vi "ml.vi"() -> ()   [LabVIEW 2014]
uses:
  ml64i4.dll
panel:
  out "Argument":string="LabVIEW"
  out "Cursor":i32
  in  "Console":string
  in  "Link":enum16{"Kernel", "Install"}(ring)=enum."Install"
  in  "ON":bool
  in  "Quit":bool
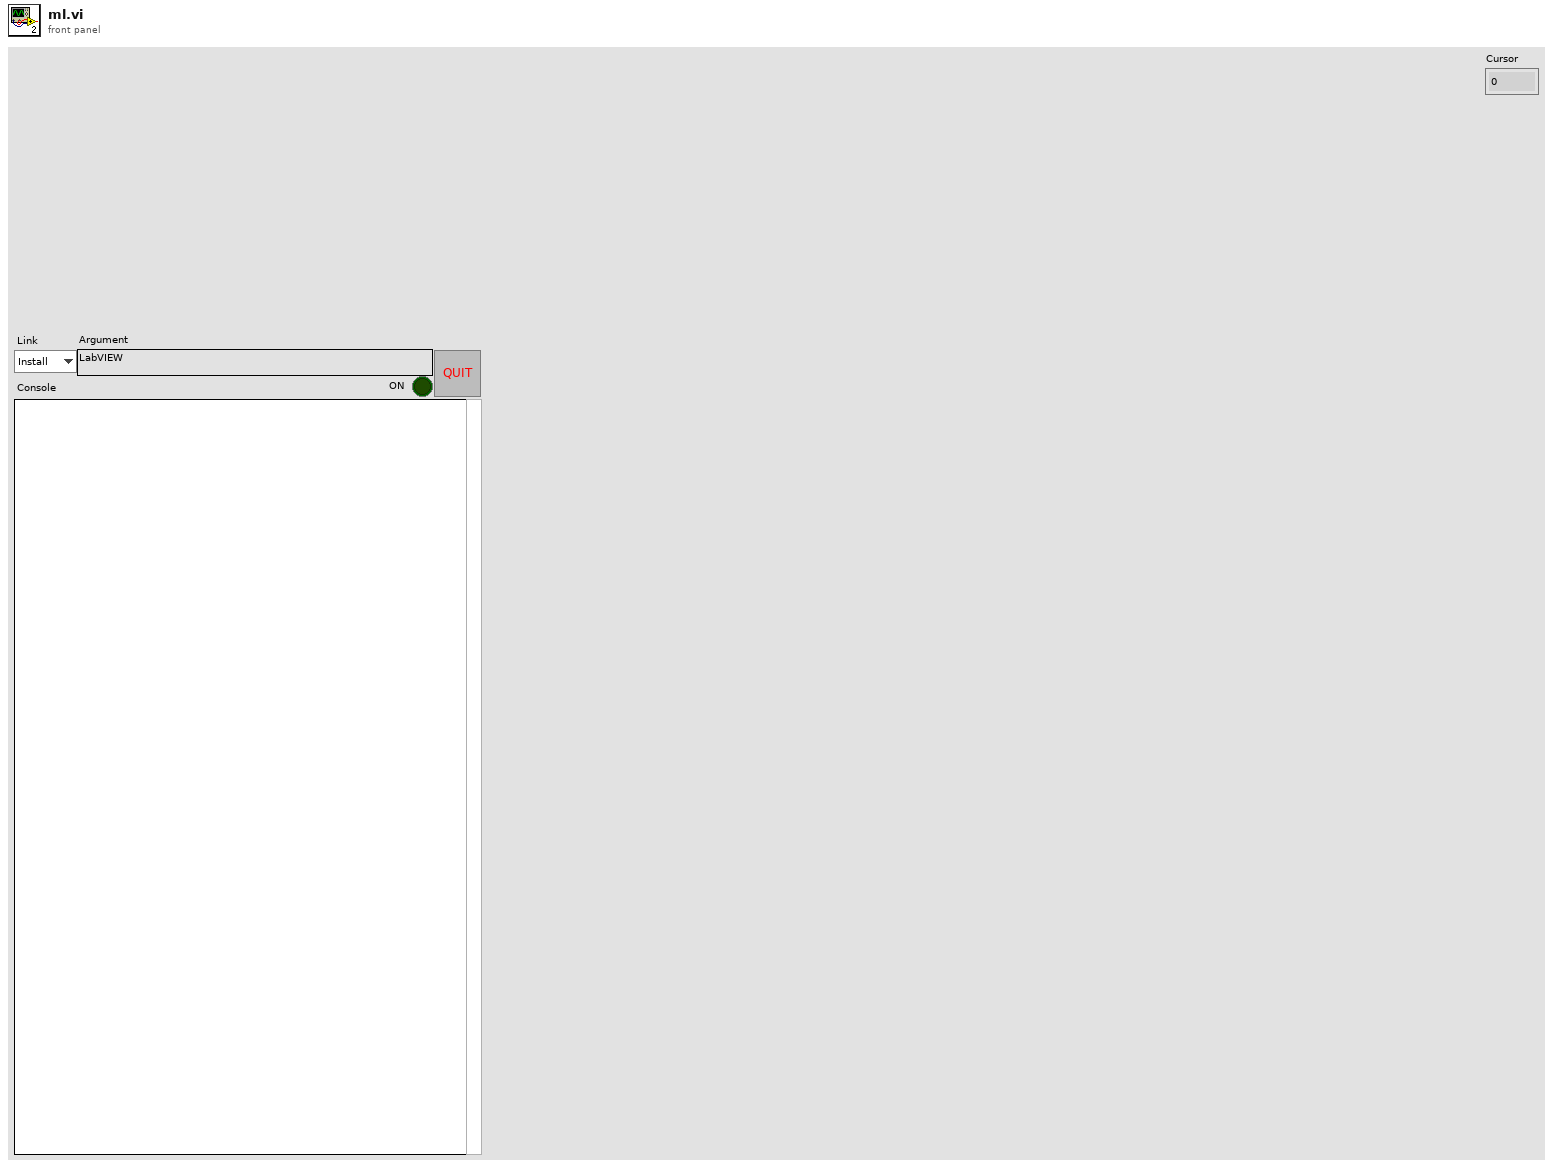
[diagram p1: front panel]
types:
  T1 = typedef "eventvkey.ctl" = enum16{"ASCII", "Enter", "Return", "Shift", "Ctrl", "Alt", "Cmd", "Opt", "Caps", "NumLock", "Clear", "Break", "Up", "Down", "Left", "Right", "Insert", "Delete", "Home", "End", "PageUp", "PageDown", "Escape", "Help", "Pause", "ScrollLock", "F1", "F2", "F3", "F4", "F5", "F6", "F7", "F8", "F9", "F10", "F11", "F12", "F13", "F14", "F15", "F16", "F17", "F18", "F19", "F20", "F21", "F22", "F23", "F24", "Play", "VolumeUp", "VolumeDown", "Mute", "Two Byte Char"}
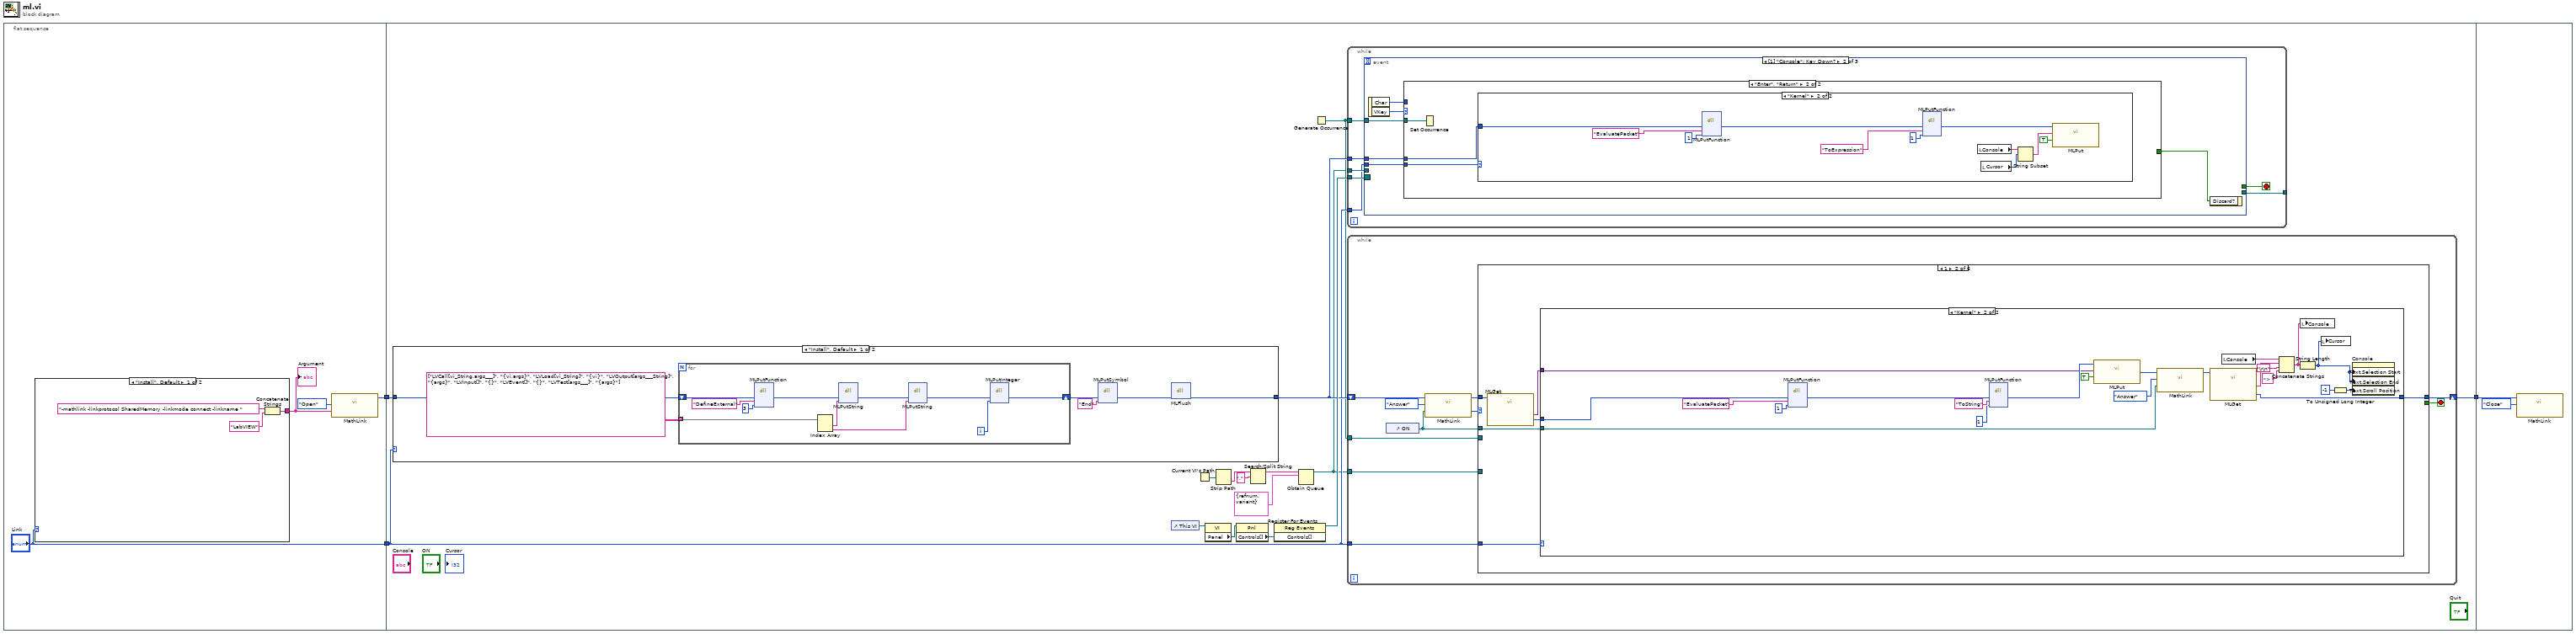
[diagram p0: block diagram]
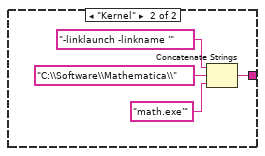
[diagram p2: hidden frame]
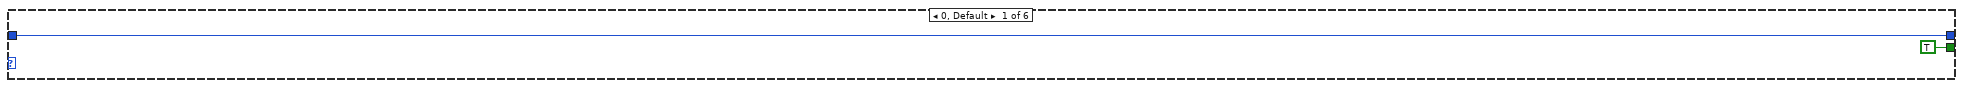
[diagram p3: hidden frame]
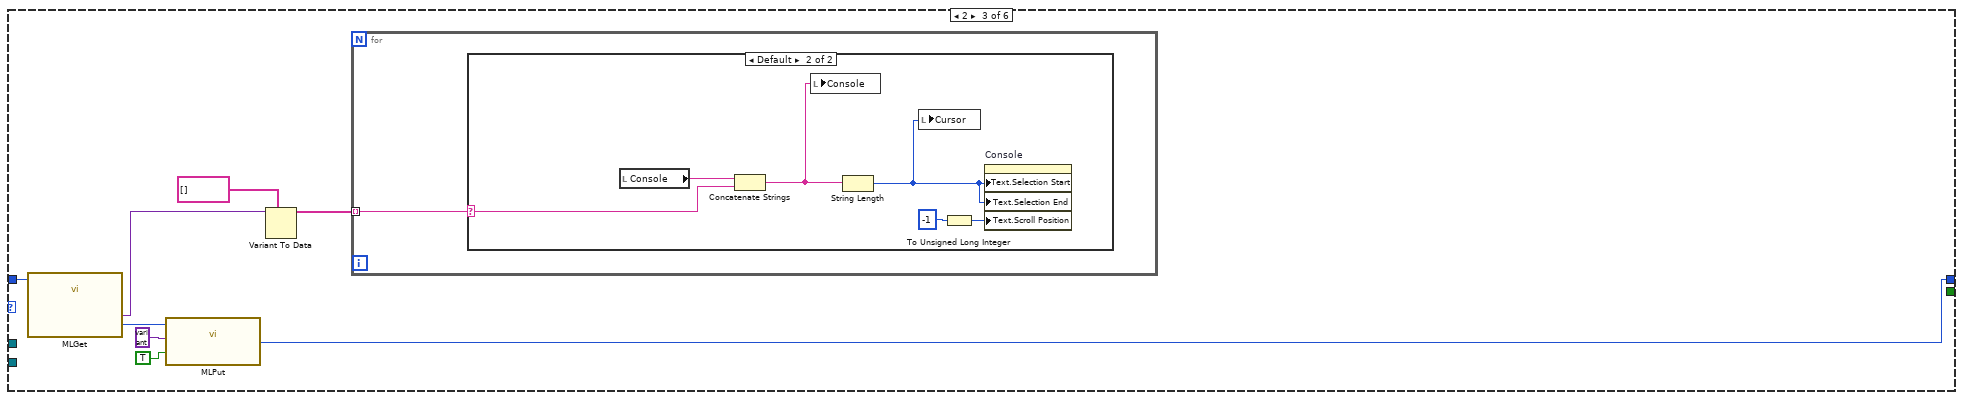
[diagram p5: hidden frame]
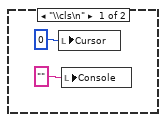
[diagram p6: hidden frame]
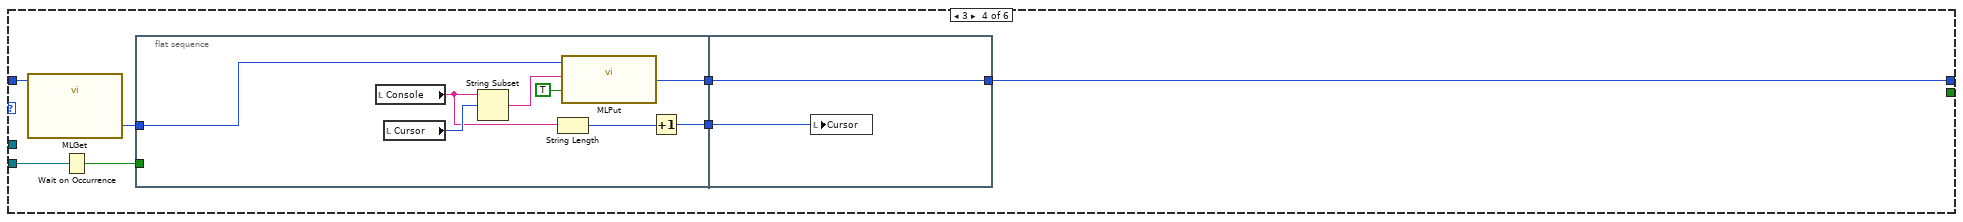
[diagram p7: hidden frame]
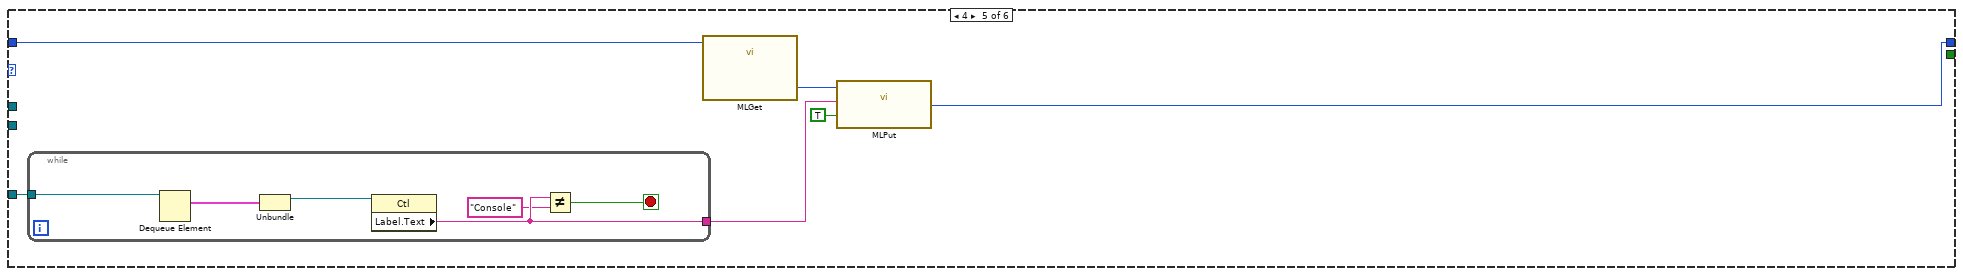
[diagram p8: hidden frame]
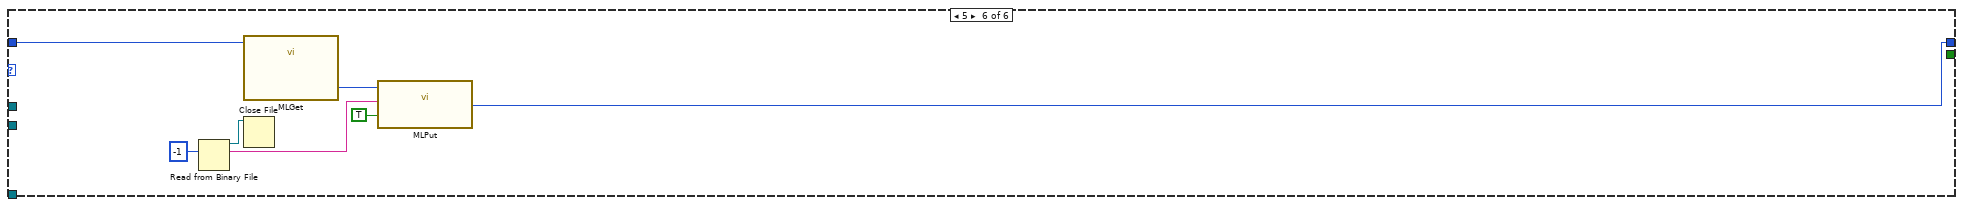
[diagram p9: hidden frame]
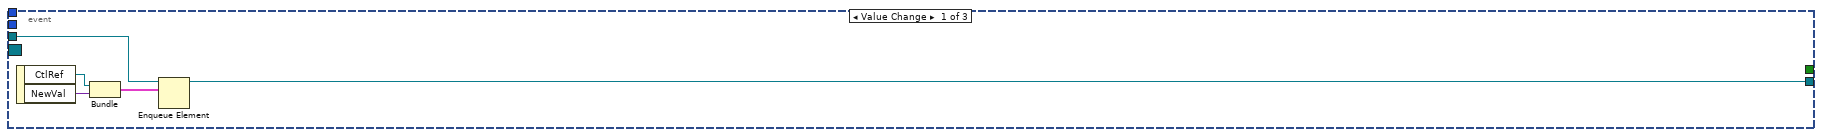
[diagram p10: hidden frame]
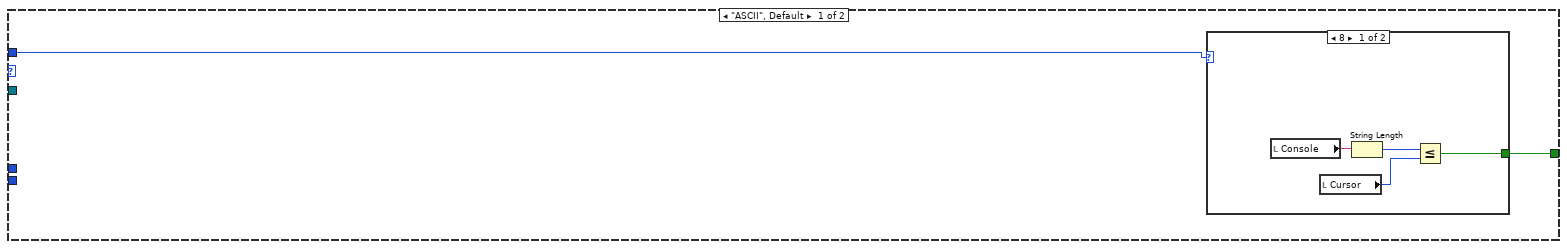
[diagram p11: hidden frame]
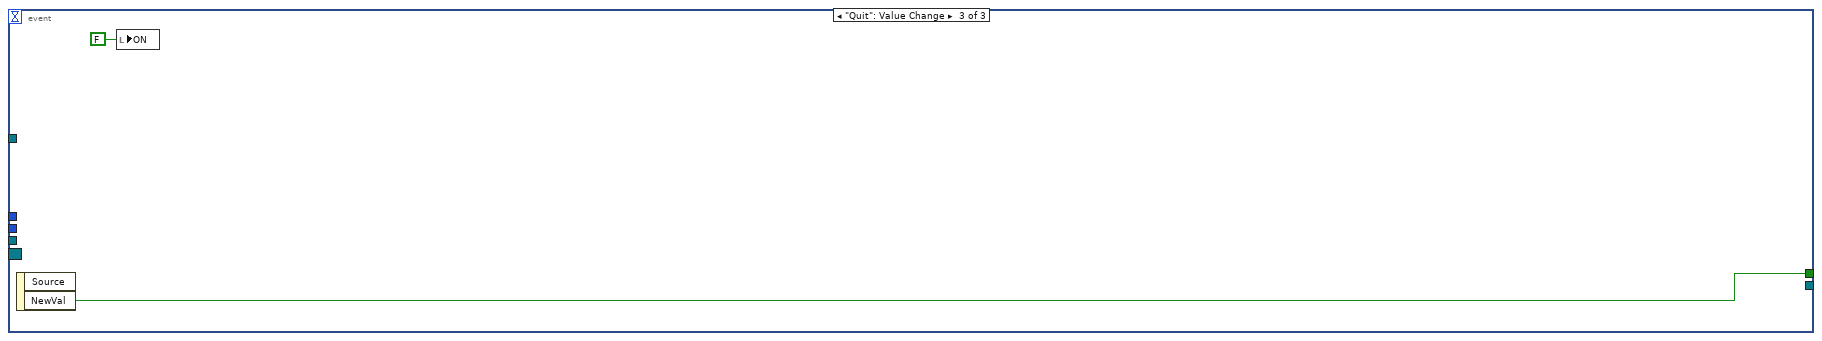
[diagram p14: hidden frame]
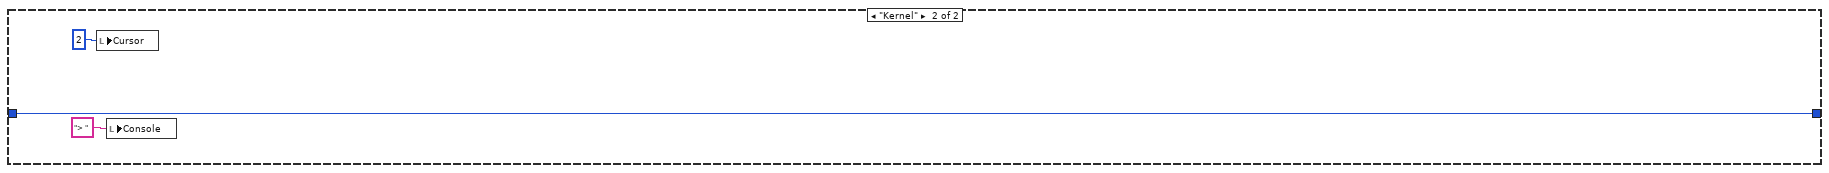
[diagram p15: hidden frame]
diagram:
  n1 = flat-sequence {
    tunnel: [w6] -> w3
    tunnel: ["Link"] -> w1
    tunnel: w3 -> [w20]
    tunnel: [w19] -> w2
    tunnel: w1 -> [w17]
    tunnel: w2 -> [w184]
    frame #0 {
      n2 = case shown="\"Install\", Default" "Link" {
        tunnel: [w9 w11] -> w4
        frame "Install", Default {
          n3 = Concatenate Strings("-mathlink -linkprotocol SharedMemory -linkmode connect -linkname ", "LabVIEW" ("string")) -> (w9:string)
        }
        frame "Kernel" {
          n4 = Concatenate Strings("-linklaunch -linkname '" ("string"), "C:\\Software\\Mathematica\\" ("string"), "math.exe'" ("string")) -> (w11:string)
        }
      }
      "Argument" <- w4
      n5 = call "MathLink.vi"("Arg"=w4, "Action"=enum16{"Open", "Answer", "Close"}."Open") -> ("mlp out"=w6:u64)  [unwired: 1 in, 1 out]
    }
    frame #1 {
      n6 = case shown="\"Install\", Default" w17 {
        tunnel: w20 -> [w164 w181]
        tunnel: [w166 w181] -> w18
        frame "Install", Default {
          n7 = for {
            shift-right: [w178] -> w169
            shift-left: w164 -> [w171]
            tunnel: string[][] [["LVCall[vi_String,args___]", "{vi,args}"], ["LVLoad[vi_String]", "{vi}"], ["LVOutput[args___String]", "{args}"], ["LVInput[]", "{}"], ["LVEvent[]", "{}"], ["LVTest[args___]", "{args}"]] -> [w177] mode=indexing
            i -> [w174]
            n8 = dll-call lib="ml64i4.dll" fn="MLPutFunction"("mlp"=w171, "s"="DefineExternal", "argc"=3) -> ("mlp"=w170:u64)  [unwired: 6 in, 2 out]
            n9 = Index Array(array=w177) -> (element #1=w176:string, element #2=w175:string)  [unwired: 2 in]
            n10 = dll-call lib="ml64i4.dll" fn="MLPutString"("mlp"=w170, "s"=w176) -> ("mlp"=w180:u64)  [unwired: 5 in, 2 out]
            n11 = dll-call lib="ml64i4.dll" fn="MLPutString"("mlp"=w180, "s"=w175) -> ("mlp"=w179:u64)  [unwired: 5 in, 2 out]
            n12 = dll-call lib="ml64i4.dll" fn="MLPutInteger"("mlp"=w179, "i"=w174) -> ("mlp"=w178:u64)  [unwired: 5 in, 2 out]
          }
          n13 = dll-call lib="ml64i4.dll" fn="MLPutSymbol"("mlp"=w169, "s"="End") -> ("mlp"=w167:u64)  [unwired: 5 in, 2 out]
          n14 = dll-call lib="ml64i4.dll" fn="MLFlush"("mlp"=w167) -> ("mlp"=w166:u64)  [unwired: 4 in, 2 out]
        }
        frame "Kernel" {
          n15 = local write "Cursor"(2 ("Cursor")) -> ()
          n16 = local write "Console"("> " ("Console")) -> ()
        }
      }
      n17 = control-ref of="This VI"() -> (w28:refnum<vi>)
      n18 = Current VI's Path() -> (path=w22:path)
      n19 = property class="VI"(reference=w28) -> ("Panel"=w29:refnum<vi>)  [unwired: 1 in, 2 out]
      n20 = Strip Path(path=w22) -> (name=w23:string)  [unwired: 1 out]
      n21 = property class="Pnl"(reference=w29) -> ("Controls[]"=w27:refnum<vi>[])  [unwired: 1 in, 2 out]
      n22 = Search/Split String(string=w23, search string/char (-)=".") -> (substring before match=w21:string)  [unwired: 1 in, 2 out]
      n23 = register-events(w27) -> (reference out=w26:refnum<event-registration>)  [unwired: 2 in, 1 out]
      n24 = Obtain Queue(name (unnamed)=w21, element data type=cluster{"CtlRef":refnum<vi>, "NewVal":variant} {"CtlRef"=refnum, "NewVal"=variant} ("output cluster")) -> (queue out=w15:refnum<queue>)  [unwired: 3 in, 2 out]
      n25 = Generate Occurrence() -> (w16:refnum<k4>)
      n26 = while {
        tunnel: w15 -> [w130]
        tunnel: w26 -> [w129]
        tunnel: [w128] -> _
        tunnel: w16 -> [w126]
        tunnel: w18 -> [w125]
        tunnel: w17 -> [w124]
        stop <- w127 stop-if-true
        n27 = event shown="[1] \"Console\": Key Down?" {
          selector: w129 -> [_ _ _]
          dyn-events: _ -> [_ _ _]
          timeout: _ -> [_ _ _]
          tunnel: w130 -> [w135 _ _]
          tunnel: [w132 _ _] -> w128
          tunnel: [_ _ w163] -> w127
          tunnel: w126 -> [_ w139 _]
          tunnel: w125 -> [_ w137 _]
          tunnel: w124 -> [_ w136 _]
          event Value Change {
            n28 = event-data() -> ("CtlRef"=w131:refnum<vi>, "NewVal"=w134:variant)  [unwired: 1 in]
            n29 = Bundle("CtlRef"=w131, "NewVal"=w134) -> (w133:cluster{"CtlRef":refnum<vi>, "NewVal":variant})  [unwired: 1 in]
            n30 = Enqueue Element(queue=w135, element=w133) -> (queue out=w132:refnum<queue>)  [unwired: 2 in, 2 out]
          }
          event "Console": Key Down? {
            n31 = event-data() -> ("Char"=w140:i16, "VKey"=w141:T1)  [unwired: 1 in]
            n32 = case shown="\"Enter\", \"Return\"" w141 {
              tunnel: w140 -> [w143 _]
              tunnel: [w142 _] -> w138
              tunnel: w139 -> [_ w150]
              tunnel: w137 -> [_ w149]
              tunnel: w136 -> [_ w148]
              frame "ASCII", Default {
                n33 = case shown="8" w143 {
                  tunnel: [w145 _] -> w142
                  frame 8 {
                    n34 = local read "Console"() -> (w144:string)
                    n35 = local read "Cursor"() -> (w146:i32)
                    n36 = String Length(string=w144) -> (length=w147:i32)
                    n37 = Less Or Equal?(x=w147, y=w146) -> (x <= y?=w145:bool)
                  }
                  frame Default {
                  }
                }
              }
              frame "Enter", "Return" {
                n38 = Set Occurrence(w150) -> ()
                n39 = case shown="\"Kernel\"" w148 {
                  tunnel: w149 -> [_ w154]
                  frame "Install", Default {
                  }
                  frame "Kernel" {
                    n40 = dll-call lib="ml64i4.dll" fn="MLPutFunction"("mlp"=w154, "s"="EvaluatePacket", "argc"=1) -> ("mlp"=w160:u64)  [unwired: 6 in, 2 out]
                    n41 = dll-call lib="ml64i4.dll" fn="MLPutFunction"("mlp"=w160, "s"="ToExpression", "argc"=1) -> ("mlp"=w159:u64)  [unwired: 6 in, 2 out]
                    n42 = local read "Console"() -> (w151:string)
                    n43 = local read "Cursor"() -> (w152:i32)
                    n44 = String Subset(string=w151, offset (0)=w152) -> (substring=w155:string)  [unwired: 1 in]
                    n45 = call "MLPut.vi"("End"=TRUE, "Variant"=w155, "mlp in"=w159) -> ()  [unwired: 1 out]
                  }
                }
              }
            }
            n46 = event-data("Discard?"=w138) -> ()  [unwired: 1 in, 1 out]
          }
          event "Quit": Value Change {
            n47 = event-data() -> ("NewVal"=w163:bool)  [unwired: 1 in, 1 out]
            n48 = local write "ON"(FALSE ("MathLink")) -> ()
          }
        }
      }
      n49 = while {
        shift-right: [w35] -> w19
        shift-left: w18 -> [w39]
        tunnel: w17 -> [w32]
        tunnel: w16 -> [w31]
        tunnel: w15 -> [w30]
        stop <- w37 stop-if-true
        n50 = control-ref of="ON"() -> (w33:refnum<vi>)
        n51 = call "MathLink.vi"("Arg"=w33, "Action"=enum16{"Open", "Answer", "Close"}."Answer", "mlp in"=w39) -> ("Status"=w38:i32, "mlp out"=w36:u64)
        n52 = case shown="1" w38 {
          tunnel: [TRUE ("End") _ _ _ _ _] -> w37
          tunnel: w36 -> [w40 w47 w78 w91 w106 w121]
          tunnel: [w40 w44 w74 w92 w107 w118] -> w35
          tunnel: w33 -> [_ w43 _ _ _ _]
          tunnel: w32 -> [_ w42 _ _ _ _]
          tunnel: w31 -> [_ _ _ w93 _ _]
          tunnel: w30 -> [_ _ _ _ w110 _]
          frame 0, Default {
          }
          frame 1 {
            n53 = call "MLGet.vi"("mlp in"=w47) -> ("mlp out"=w46:u64, "Variant"=w45:variant)  [unwired: 1 in, 4 out]
            n54 = case shown="\"Kernel\"" w42 {
              tunnel: w46 -> [w48 w64]
              tunnel: w45 -> [_ w63]
              tunnel: [w48 w62] -> w44
              tunnel: w43 -> [_ w58]
              frame "Install", Default {
              }
              frame "Kernel" {
                n55 = dll-call lib="ml64i4.dll" fn="MLPutFunction"("mlp"=w64, "s"="EvaluatePacket", "argc"=1) -> ("mlp"=w69:u64)  [unwired: 6 in, 2 out]
                n56 = dll-call lib="ml64i4.dll" fn="MLPutFunction"("mlp"=w69, "s"="ToString", "argc"=1) -> ("mlp"=w66:u64)  [unwired: 6 in, 2 out]
                n57 = call "MLPut.vi"("End"=TRUE, "Variant"=w63, "mlp in"=w66) -> ("mlp out"=w60:u64)
                n58 = call "MathLink.vi"("Arg"=w58, "Action"=enum16{"Open", "Answer", "Close"}."Answer", "mlp in"=w60) -> ("mlp out"=w57:u64)  [unwired: 1 out]
                n59 = call "MLGet.vi"("mlp in"=w57) -> ("mlp out"=w62:u64, "String"=w55:string)  [unwired: 1 in, 4 out]
                n60 = local read "Console"() -> (w56:string)
                n61 = Concatenate Strings(w56, w55, "\r\n", "> " ("string")) -> (w53:string)
                n62 = local write "Console"(w53) -> ()
                n63 = String Length(string=w53) -> (length=w50:i32)
                n64 = local write "Cursor"(w50) -> ()
                n65 = To Unsigned Long Integer(number=-1 ("Text.Scroll Position")) -> (unsigned 32bit integer=w52:u32)
                n66 = property on="Console" class="Str"("Text.Selection Start"=w50, "Text.Selection End"=w50, "Text.Scroll Position"=w52) -> ()  [unwired: 2 in, 2 out]
              }
            }
          }
          frame 2 {
            n67 = call "MLGet.vi"("mlp in"=w78) -> ("mlp out"=w77:u64, "Variant"=w73:variant)  [unwired: 1 in, 4 out]
            n68 = call "MLPut.vi"("End"=TRUE, "Variant"=variant, "mlp in"=w77) -> ("mlp out"=w74:u64)
            n69 = Variant To Data(type=string[] [], Variant=w73) -> (data=w71:string[])  [unwired: 1 in, 1 out]
            n70 = for {
              tunnel: w71 -> [w79] mode=indexing
              n71 = case shown="Default" w79 {
                selector: w79 -> [_ w82]
                frame "\\cls\n" {
                  n72 = local write "Cursor"(0 ("Cursor")) -> ()
                  n73 = local write "Console"("" ("Console")) -> ()
                }
                frame Default {
                  n74 = local read "Console"() -> (w87:string)
                  n75 = Concatenate Strings(w87, w82) -> (w86:string)
                  n76 = local write "Console"(w86) -> ()
                  n77 = String Length(string=w86) -> (length=w83:i32)
                  n78 = local write "Cursor"(w83) -> ()
                  n79 = To Unsigned Long Integer(number=-1 ("Text.Scroll Position")) -> (unsigned 32bit integer=w85:u32)
                  n80 = property on="Console" class="Str"("Text.Selection Start"=w83, "Text.Selection End"=w83, "Text.Scroll Position"=w85) -> ()  [unwired: 2 in, 2 out]
                }
              }
            }
          }
          frame 3 {
            n81 = call "MLGet.vi"("mlp in"=w91) -> ("mlp out"=w90:u64)  [unwired: 1 in, 5 out]
            n82 = Wait on Occurrence(2:w93) -> (0:w94:bool)  [unwired: 2 in]
            n83 = flat-sequence {
              tunnel: w94 -> [_]
              tunnel: w90 -> [w99]
              tunnel: [w98] -> w89
              tunnel: [w95] -> w88
              tunnel: [w104] -> w92
              tunnel: w89 -> [w104]
              tunnel: w88 -> [w103]
              frame #0 {
                n84 = local read "Console"() -> (w96:string)
                n85 = local read "Cursor"() -> (w102:i32)
                n86 = String Subset(string=w96, offset (0)=w102) -> (substring=w101:string)  [unwired: 1 in]
                n87 = String Length(string=w96) -> (length=w97:i32)
                n88 = call "MLPut.vi"("End"=TRUE, "Variant"=w101, "mlp in"=w99) -> ("mlp out"=w98:u64)
                n89 = Increment(x=w97) -> (x+1=w95:i32)
              }
              frame #1 {
                n90 = local write "Cursor"(w103) -> ()
              }
            }
          }
          frame 4 {
            n91 = while {
              tunnel: w110 -> [w116]
              tunnel: [w113] -> w109
              stop <- w111 stop-if-true
              n92 = Dequeue Element(queue=w116) -> (element=w115:cluster{"CtlRef":refnum<vi>, "NewVal":variant})  [unwired: 2 in, 3 out]
              n93 = Unbundle(w115) -> ("CtlRef"=w114:refnum<vi>)  [unwired: 1 out]
              n94 = property class="Ctl"(reference=w114) -> ("Label.Text"=w113:string)  [unwired: 1 in, 2 out]
              n95 = Not Equal?(x=w113, y="Console") -> (x != y?=w111:bool)
            }
            n96 = call "MLGet.vi"("mlp in"=w106) -> ("mlp out"=w105:u64)  [unwired: 1 in, 5 out]
            n97 = call "MLPut.vi"("End"=TRUE, "Variant"=w109, "mlp in"=w105) -> ("mlp out"=w107:u64)
          }
          frame 5 {
            n98 = Read from Binary File(10:-1 ("count (1)")) -> (2:w120:string, 3:w122:refnum<file>)  [unwired: 5 in, 2 out]
            n99 = call "MLGet.vi"("mlp in"=w121) -> ("mlp out"=w117:u64)  [unwired: 1 in, 5 out]
            n100 = Close File(refnum=w122) -> ()  [unwired: 1 in, 2 out]
            n101 = call "MLPut.vi"("End"=TRUE, "Variant"=w120, "mlp in"=w117) -> ("mlp out"=w118:u64)
          }
        }
      }
    }
    frame #2 {
      n102 = call "MathLink.vi"("Action"=enum16{"Open", "Answer", "Close"}."Close", "mlp in"=w184) -> ()  [unwired: 1 in, 2 out]
    }
  }
